vi "W&R(Know Size Compare Check With Data).vi"(0 "VISA resource name in":refnum<visa-resource-name>, 5 "写入指令/数据":string, 7 "总字节数":u32, 9 "超时":u32=1000, 11 "error in":errorcluster, 12 "比较校验":string) -> (4 "VISA resource name out":refnum<visa-resource-name>, 6 "读取缓冲区":string, 15 "error out":errorcluster)   [LabVIEW 2020]
uses:
  <vilib>/Instr/_visa.llb/VISA Set IO Buffer Mask.ctl
  <vilib>/Instr/_visa.llb/VISA Flush IO Buffer Mask.ctl
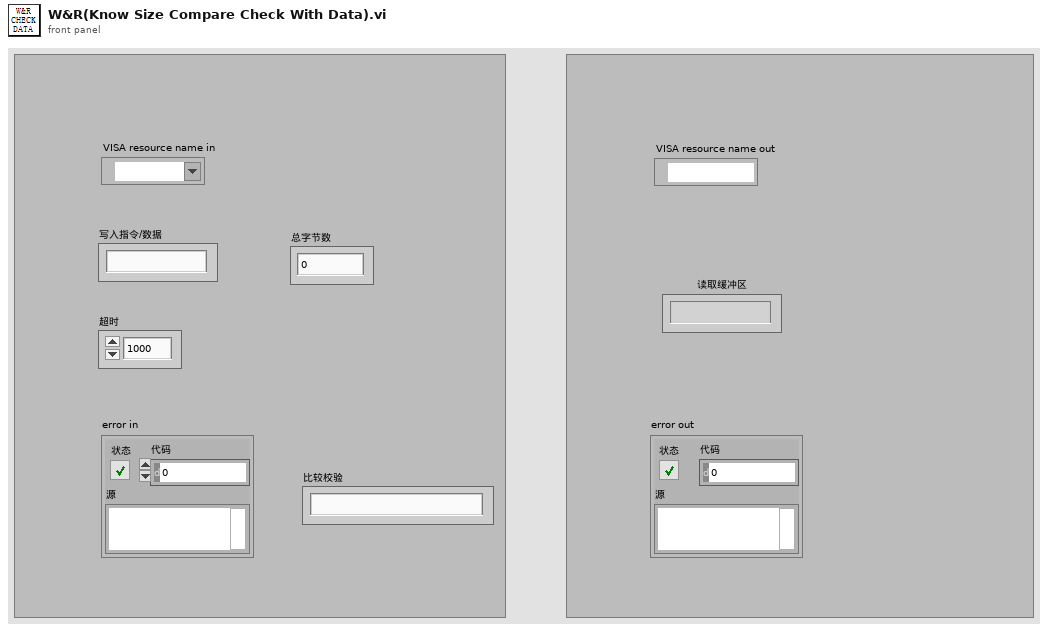
[diagram p1: front panel]
types:
  T1 = typedef "VISA Flush IO Buffer Mask.ctl" = u16
  T2 = typedef "VISA Set IO Buffer Mask.ctl" = u16
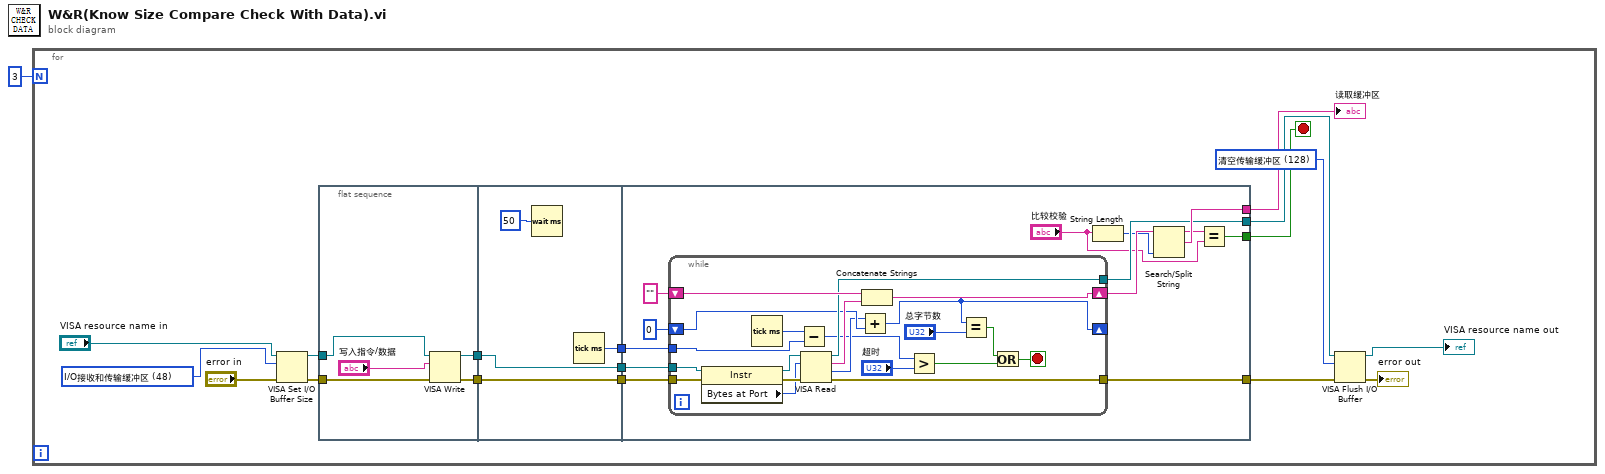
[diagram p0: block diagram]
diagram:
  n1 = for {
    N: 3 -> [_]
    stop <- w13 stop-if-true
    w6 = T1 128 items=["清空接收缓冲区"=16, "向设备写入传输缓冲区"=32, "清空接收缓冲区（无I/O）"=64, "清空传输缓冲区"=128] ("Mask")
    w11 = T2 48 items=["I/O接收缓冲区"=16, "I/O传输缓冲区"=32, "I/O接收和传输缓冲区"=48] ("Mask")
    n2 = VISA Set I/O Buffer Size(VISA resource name="VISA resource name in", mask (16)=w11, error in (no error)="error in") -> (VISA resource name out=w9:refnum<visa-resource-name>, error out=w7:errorcluster)  [unwired: 1 in]
    n3 = flat-sequence {
      tunnel: w9 -> [w23]
      tunnel: [w22] -> w18
      tunnel: [w20] -> w17
      tunnel: w7 -> [w19]
      tunnel: [w27] -> w16
      tunnel: w18 -> [w27]
      tunnel: [w26] -> w15
      tunnel: w17 -> [w26]
      tunnel: [w25] -> w12
      tunnel: w16 -> [w40]
      tunnel: w15 -> [w39]
      tunnel: [w37] -> w13
      tunnel: [w36] -> w14
      tunnel: [w35] -> w5
      tunnel: [w34] -> w3
      tunnel: w12 -> [w30]
      frame #0 {
        n4 = VISA Write(VISA resource name=w23, write buffer="写入指令/数据", error in (no error)=w19) -> (VISA resource name out=w22:refnum<visa-resource-name>, error out=w20:errorcluster)  [unwired: 1 out]
      }
      frame #1 {
        n5 = Wait (ms)(milliseconds to wait=u32 50 ("等待时间（毫秒）")) -> ()  [unwired: 1 out]
        n6 = Tick Count (ms)() -> (millisecond timer value=w25:u32)
      }
      frame #2 {
        n7 = while {
          tunnel: w40 -> [w61]
          tunnel: w39 -> [w60]
          shift-right: [w57] -> w38
          shift-left: "" -> [w56]
          tunnel: [w55] -> w35
          tunnel: [w54] -> w34
          shift-right: [w50] -> _
          shift-left: u32 0 -> [w51]
          tunnel: w30 -> [w46]
          stop <- w42 stop-if-true
          n8 = property class="Instr"(reference=w61, error in=w60) -> (reference out=w59:refnum<visa-resource-name>, error out=w58:errorcluster, "Bytes at Port"=w52:u32)
          n9 = Tick Count (ms)() -> (millisecond timer value=w47:u32)
          n10 = Subtract(x=w47, y=w46) -> (x-y=w45:u32)
          n11 = VISA Read(VISA resource name=w59, byte count=w52, error in (no error)=w58) -> (VISA resource name out=w55:refnum<visa-resource-name>, read buffer=w53:string, return count=w48:u32, error out=w54:errorcluster)
          n12 = Add(x=w48, y=w51) -> (x+y=w50:u32)
          n13 = Concatenate Strings(w56, w53) -> (w57:string)
          n14 = Greater?(x=w45, y="超时") -> (0:w43:bool)
          n15 = Equal?(x=w50, y="总字节数") -> (x = y?=w44:bool)
          n16 = Or(x=w44, y=w43) -> (x .or. y?=w42:bool)
        }
        n17 = String Length(string="比较校验") -> (length=w28:i32)
        n18 = Search/Split String(string=w38, offset (0)=w28) -> (substring before match=w29:string, match + rest of string=w36:string)  [unwired: 1 in, 1 out]
        n19 = Equal?(x=w29, y="比较校验") -> (x = y?=w37:bool)
      }
    }
    n20 = VISA Flush I/O Buffer(VISA resource name=w5, mask (16)=w6, error in (no error)=w3) -> (VISA resource name out=→"VISA resource name out":refnum<visa-resource-name>, error out=→"error out":errorcluster)
    "读取缓冲区" <- w14
  }
